vi "DeQ_Calibrator_QMH.vi"(8 "Error In":errorcluster, 11 "Queue In":refnum<queue>) -> (0 "Error Out":errorcluster, 1 "Message":variant, 2 "Instruction":T1, 3 "Queue Out":refnum<queue>)   [LabVIEW 2021, in "Queues.lvlib"]
doc: "This subVI is used to dequeue and unbundle the elements of DaQ QMH queue."
uses:
  Queues.lvlib
  Tipski Definicii/Kalibrator_Sostojbi.ctl
panel:
  # "Input"
  # "Output"
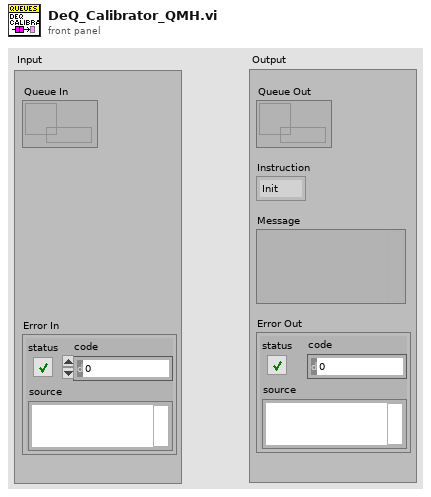
[diagram p1: front panel]
types:
  T1 = typedef "Kalibrator_Sostojbi.ctl" = enum16{"Init", "Idle", "Standby", "Operate ", "End"}
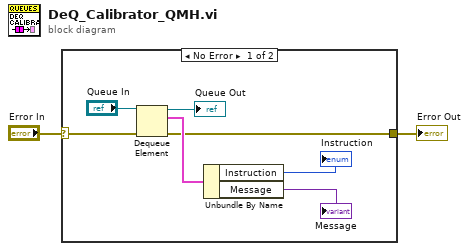
[diagram p0: block diagram]
diagram:
  n1 = case shown="No Error" "Error In" {
    selector: "Error In" -> [w6 w10]
    tunnel: [w5 w10] -> w1
    frame No Error {
      n2 = Dequeue Element(queue="Queue In", error in (no error)=w6) -> (queue out=→"Queue Out":refnum<queue>, element=w9:cluster{"Instruction":T1, "Message":variant}, error out=w5:errorcluster)  [unwired: 1 in, 1 out]
      n3 = Unbundle By Name(w9) -> ("Instruction"=→"Instruction":T1, "Message"=→"Message":variant)
    }
    frame Error {
    }
  }
  "Error Out" <- w1
